vi "clase1.vi"() -> ()   [LabVIEW 2011]
panel:
  out "Multiplicar":dbl
  out "División":dbl
  out "Resta":dbl
  out "Suma":dbl
  in  "Numero2":dbl
  in  "Numero1":dbl
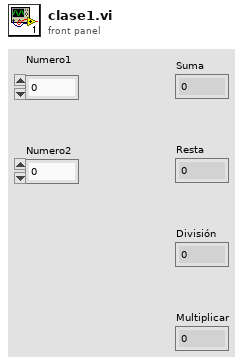
[diagram p1: front panel]
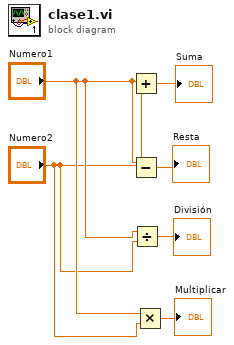
[diagram p0: block diagram]
diagram:
  n1 = Add(x="Numero1", y="Numero2") -> (x+y=→"Suma":dbl)
  n2 = Subtract(x="Numero1", y="Numero2") -> (x-y=→"Resta":dbl)
  n3 = Divide(x="Numero1", y="Numero2") -> (x/y=→"División":dbl)
  n4 = Multiply(x="Numero1", y="Numero2") -> (x*y=→"Multiplicar":dbl)
